vi "Main.vi"() -> ()   [LabVIEW 2017, in "Strategy Pattern Demo.lvclass"]
uses:
  Strategy Pattern Demo.lvclass
  Context Class/Context.lvclass
  ConsoleOut/Print Options.ctl
  OperationAdd Class/OperationAdd.lvclass
  C:/Users/fflores/Documents/LabVIEW-Open-Projects/LabIVEW OOP Design Patterns/Strategy Pattern/Strategy Class/Strategy.lvclass
  OperationMultiply Class/OperationMultiply.lvclass
  OperationSubtract Class/OperationSubtract.lvclass
panel:
  in  "Number 2":dbl
  in  "Number 1":dbl
  in  "Strategy":enum16{"Add", "Multiply", "Subtract"}(ring)
  # "1. Choose your Strategy\n2. Enter \"Number 1\" and \"Number 2\"\n3. Run the VI"
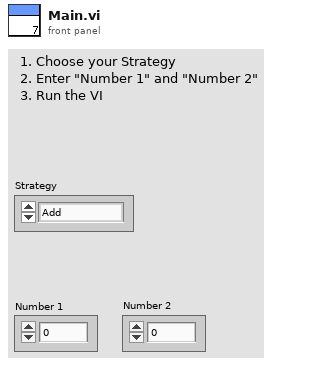
[diagram p1: front panel]
types:
  T1 = typedef "Print Options.ctl" = enum16{"Create", "Get Reference", "Print", "Print Header", "Close"}
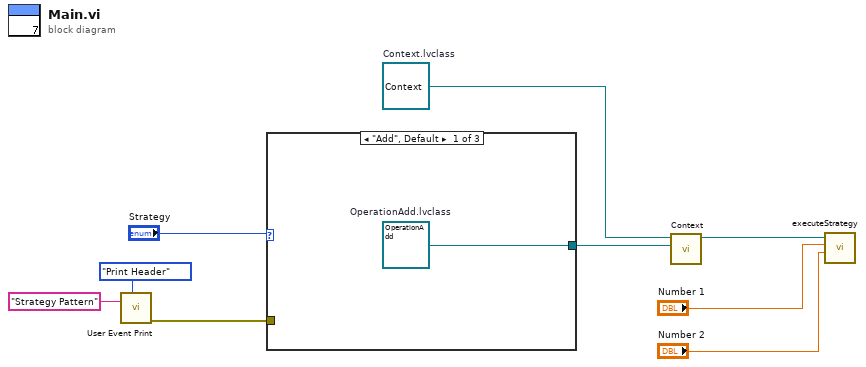
[diagram p0: block diagram]
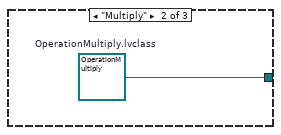
[diagram p2: hidden frame]
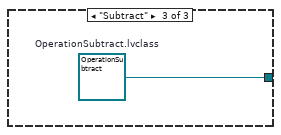
[diagram p3: hidden frame]
diagram:
  w7 = refnum<class "Context.lvclass"> refnum  # Context.lvclass
  n1 = call "User Event Print.vi"("Options"=Print_Options."Print Header", "String to Print"="Strategy Pattern") -> ("error out"=w1:errorcluster)  [unwired: 8 in, 1 out]
  n2 = case shown="\"Add\", Default" "Strategy" {
    tunnel: [w10 w11 w12] -> w8
    tunnel: w1 -> [_ _ _]
    frame "Add", Default {
      w10 = refnum<class "OperationAdd.lvclass"> refnum  # OperationAdd.lvclass
    }
    frame "Multiply" {
      w11 = refnum<class "OperationMultiply.lvclass"> refnum  # OperationMultiply.lvclass
    }
    frame "Subtract" {
      w12 = refnum<class "OperationSubtract.lvclass"> refnum  # OperationSubtract.lvclass
    }
  }
  n3 = call "Context.vi"("Strategy.lvclass"=w8, "Context in"=w7) -> ("Context out"=w6:refnum<class "Context.lvclass">)  [unwired: 8 in, 1 out]
  n4 = call "executeStrategy.vi"("num2"="Number 2", "num1"="Number 1", "Context in"=w6) -> ()  [unwired: 7 in, 2 out]
